vi "HMI Pop Up Alpha KB.vi"(4 "Password Display (F)":bool, 5 "Hide OVR Key (T)":bool, 6 "Max Length (70)":i32=70, 8 "error in (no error)":errorcluster, 10 "String In":string, 11 "Message In":string) -> (0 "error out":errorcluster, 1 "Canceled":bool, 2 "String Out":string)   [LabVIEW 2015]
doc: "Name: Pop Up Keyboard\nAuthor: Georges Janveau, Columbia Forest Products\n\nDESCRIPTION\nSimulates an alphanumeric keyboard intended to be used on a touchscreen PC. The input control can be set for standard or password display. The OVR key can be shown or hidden.\n\nINPUTS\nMessage In - Optional message displayedin the title bar.\nString In - Sets the initial value of the edit box.\nPassword Display (F) - Sets standard or password display.\nHide OVR Key (T) - Hides or displays the OVR key button.\nMax Length (255) - Sets the maximum length allowed in the edit box.\n\nOUTPUTS\nString Out - Result (will contain String In if the user cancels).\nCanceled - True if the user cancels.\n\n----------------------------------------------------------------------------------------------------------------"
uses:
  srv_label_inspection_line2-3-4-5/Encoder - PLC SR - MF - Image Buffer/Version2/Src/OGN_SRV_PHC_SUBVI/OGN_SRV_PHC_UI/Keyboard/Driver Commands.ctl
panel:
  out "Caps on":bool
  in  "Shift 2":bool
  in  "<\n,":bool
  in  "?\n/":bool
  in  ">\n.":bool
  in  "M\nm":bool
  in  "N\nn":bool
  in  "B\nb":bool
  in  "V\nv":bool
  in  "C\nc":bool
  in  "X\nx":bool
  in  "Z\nz":bool
  in  "\"\n'":bool
  in  ":\n;":bool
  in  "L\nl":bool
  in  "K\nk":bool
  in  "J\nj":bool
  in  "H\nh":bool
  in  "G\ng":bool
  in  "F\nf":bool
  in  "D\nd":bool
  in  "S\ns":bool
  in  "A\na":bool
  in  "}\n]":bool
  in  "{\n[":bool
  in  "|\n\\":bool
  in  "+\n=":bool
  in  "_\n-":bool
  in  "P\np":bool
  in  "O\no":bool
  in  "I\ni":bool
  in  "U\nu":bool
  in  "Y\ny":bool
  in  "T\nt":bool
  in  "R\nr":bool
  in  "E\ne":bool
  in  "W\nw":bool
  in  ")\n0":bool
  in  "(\n9":bool
  in  "*\n8":bool
  in  "&\n7":bool
  in  "^\n6":bool
  in  "%\n5":bool
  in  "$\n4":bool
  in  "#\n3":bool
  in  "@\n2":bool
  in  "!\n1":bool
  in  "Q\nq":bool
  in  "Right":bool
  in  "Left":bool
  in  "Over Write":bool
  in  "Ok":bool
  in  "Cancel":bool
  in  "Space":bool
  in  "Shift":bool
  in  "CAPS":bool
  in  "Text":string
  in  "Backspace":bool
  # "Inputs"
  # "Outputs"
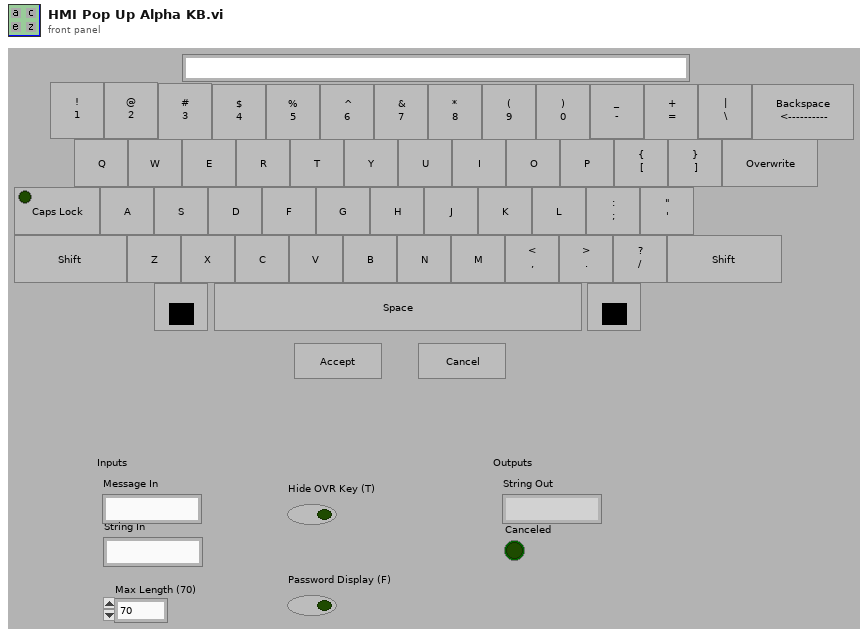
[diagram p1: front panel]
types:
  T1 = typedef "Driver Commands.ctl" = enum16{"No Command", "Initialize", "Add Character", "Replace Charcter", "Delete Character", "Move Left", "Move Right", "Update Edit Position"}
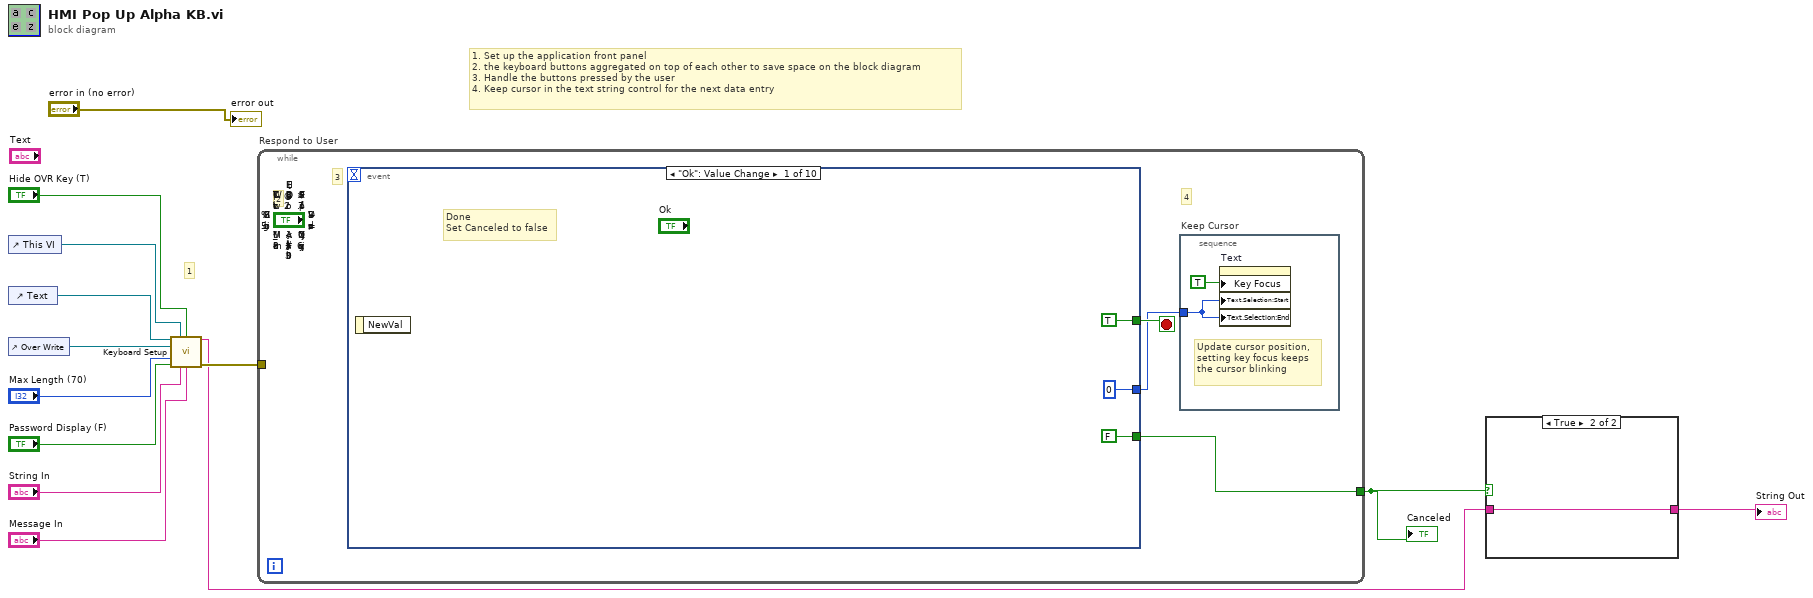
[diagram p0: block diagram]
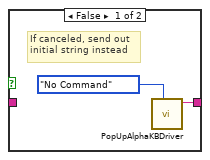
[diagram p2: hidden frame]
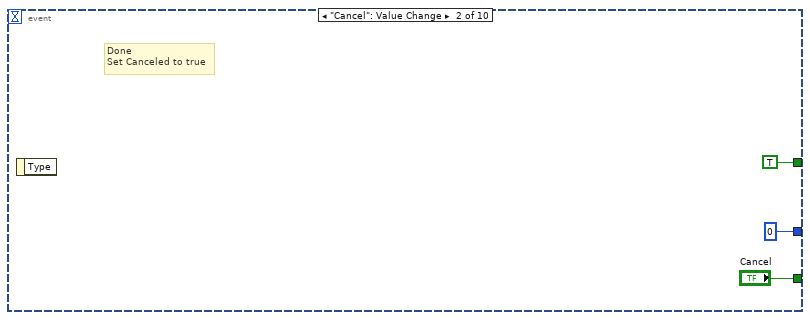
[diagram p3: hidden frame]
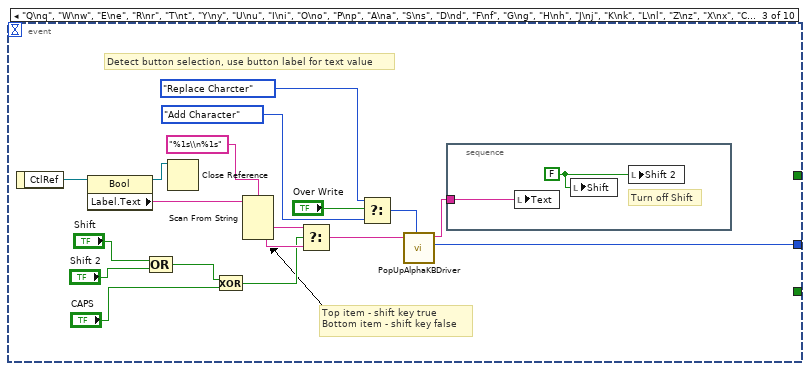
[diagram p4: hidden frame]
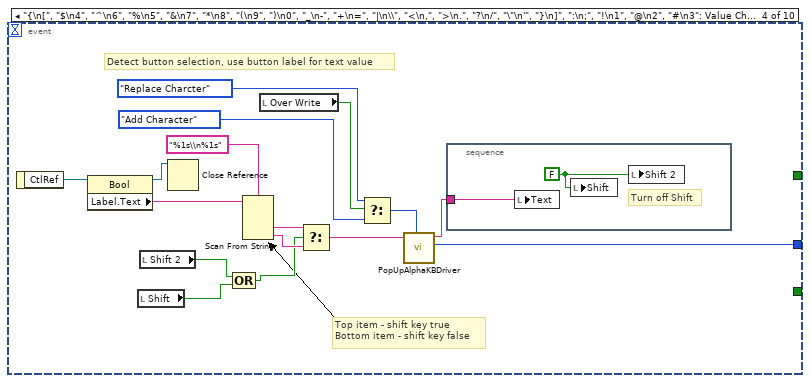
[diagram p5: hidden frame]
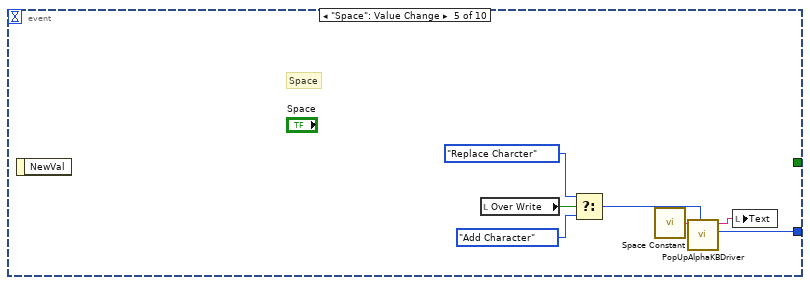
[diagram p6: hidden frame]
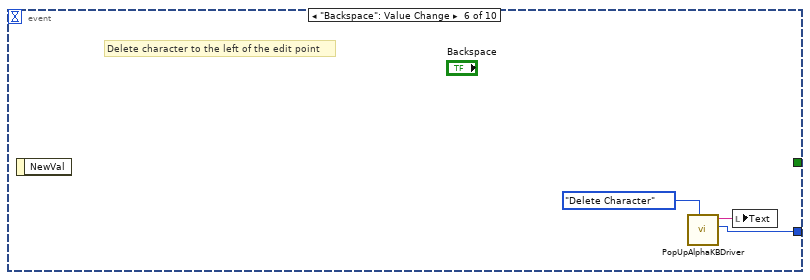
[diagram p7: hidden frame]
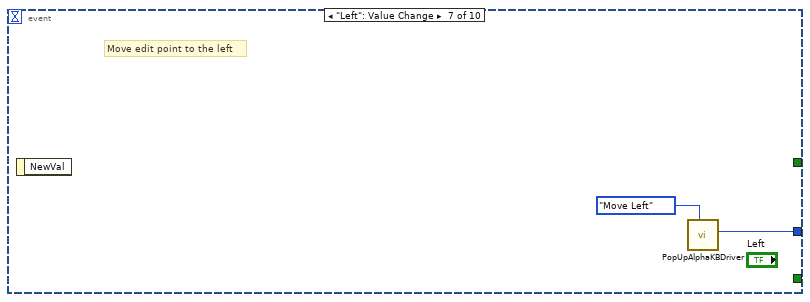
[diagram p8: hidden frame]
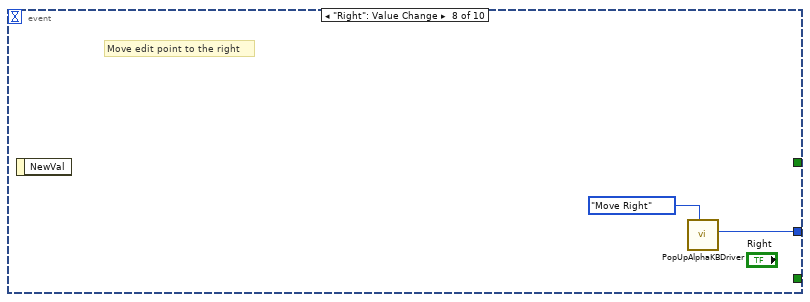
[diagram p9: hidden frame]
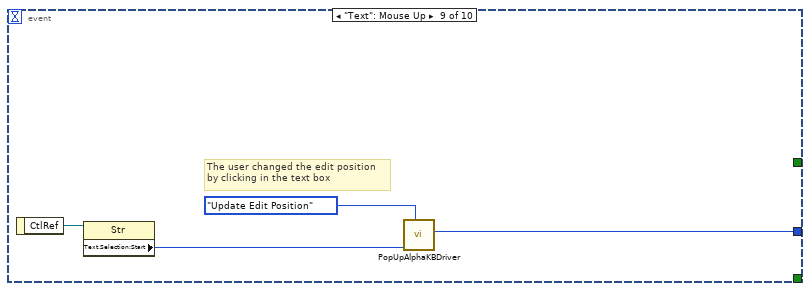
[diagram p10: hidden frame]
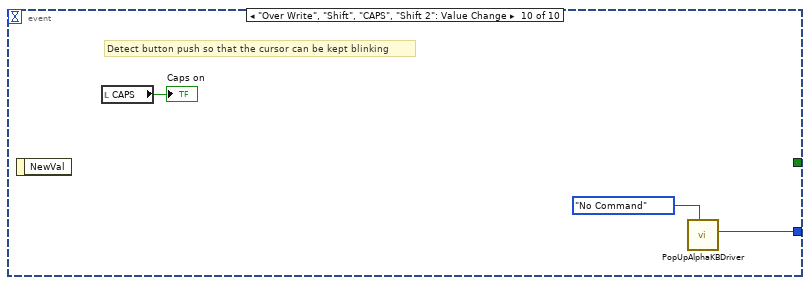
[diagram p11: hidden frame]
diagram:
  # "1. Set up the application front panel\n2. the keyboard buttons aggregated on top of each other to save space on the block diagram\n3. Handle the buttons pressed by the user\n4. Keep cursor in the text string control for the next data entry"
  # "1"
  n1 = control-ref of="This VI"() -> (w6:refnum<vi>)
  n2 = control-ref of="Text"() -> (w10:refnum<vi>)
  n3 = control-ref of="Over Write"() -> (w9:refnum<vi>)
  n4 = call "Keyboard Setup.vi"("String in"=w10, "This VI"=w6, "Hide OVR Key (T)"="Hide OVR Key (T)", "reference in"=w9, "Max Length (70)"="Max Length (70)", "Password Display (F)"="Password Display (F)", "String In"="String In", "Message In"="Message In") -> ("String Out"=w3:string, "error out"=w4:errorcluster)  [unwired: 6 in]
  n5 = while "Respond to User" {
    tunnel: [w14] -> w2
    tunnel: w4 -> [_]
    stop <- w16 stop-if-true
    # "4"
    # "2"
    # "3"
    n6 = event shown="[0] \"Ok\": Value Change" {
      selector: _ -> [_ _ _ _ _ _ _ _ _ _]
      dyn-events: _ -> [_ _ _ _ _ _ _ _ _ _]
      timeout: _ -> [_ _ _ _ _ _ _ _ _ _]
      tunnel: [TRUE TRUE _ _ _ _ _ _ _ _] -> w16
      tunnel: [0 ("Edit Position") 0 ("Edit Position") w32 w50 w65 w71 w74 w75 w77 w82] -> w15
      tunnel: [FALSE ("Cancel") "Cancel" _ _ _ _ _ _ _ _] -> w14
      event "Ok": Value Change {
        # "Done\nSet Canceled to false"
        n7 = event-data() -> ()  [unwired: 1 in, 1 out]
      }
      event "Cancel": Value Change {
        # "Done\nSet Canceled to true"
        n8 = event-data() -> ()  [unwired: 1 in, 1 out]
      }
      event "Q\nq", "W\nw", "E\ne", "R\nr", "T\nt", "Y\ny", "U\nu", "I\ni", "O\no", "P\np", "A\na", "S\ns", "D\nd", "F\nf", "G\ng", "H\nh", "J\nj", "K\nk", "L\nl", "Z\nz", "X\nx", "C\nc", "V\nv", "B\nb", "N\nn", "M\nm": Value Change {
        # "Top item - shift key true\nBottom item - shift key false"
        # "Detect button selection, use button label for text value"
        n9 = event-data() -> ("CtlRef"=w39:refnum<vi>)  [unwired: 1 in]
        n10 = property class="Bool"(reference=w39) -> (reference out=w37:refnum<vi>, "Label.Text"=w38:string)  [unwired: 1 in, 1 out]
        n11 = Compound Arithmetic op=OR("Shift", "Shift 2") -> (w27:bool)
        n12 = Close Reference(reference=w37) -> ()  [unwired: 1 in, 1 out]
        n13 = Exclusive Or(1:"CAPS", 2:w27) -> (0:w25:bool)
        n14 = Scan From String(format string="%1s\\n%1s", input string=w38) -> (output 1=w41:string, output 2=w40:string)  [unwired: 4 in, 3 out]
        n15 = Select(t=w41, s=w25, f=w40) -> (s? t:f=w36:string)
        n16 = Select(t=Driver_Commands."Replace Charcter" ("Driver Commands"), s="Over Write", f=Driver_Commands."Add Character" ("Driver Commands")) -> (s? t:f=w35:T1)
        n17 = call "PopUpAlphaKBDriver.vi"("Driver Commands"=w35, "Character"=w36) -> ("Edit Position"=w32:i32, "String Out"=w30:string)  [unwired: 8 in]
        n18 = stacked-sequence {
          tunnel: w30 -> [w44]
          frame #0 {
            w43 = FALSE ("Shift")
            # "Turn off Shift"
            n19 = local write "Text"(w44) -> ()
            n20 = local write "Shift"(w43) -> ()
            n21 = local write "Shift 2"(w43) -> ()
          }
        }
      }
      event "{\n[", "$\n4", "^\n6", "%\n5", "&\n7", "*\n8", "(\n9", ")\n0", "_\n-", "+\n=", "|\n\\", "<\n,", ">\n.", "?\n/", "\"\n'", "}\n]", ":\n;", "!\n1", "@\n2", "#\n3": Value Change {
        # "Top item - shift key true\nBottom item - shift key false"
        # "Detect button selection, use button label for text value"
        n22 = event-data() -> ("CtlRef"=w57:refnum<vi>)  [unwired: 1 in]
        n23 = property class="Bool"(reference=w57) -> (reference out=w55:refnum<vi>, "Label.Text"=w56:string)  [unwired: 1 in, 1 out]
        n24 = local read "Shift"() -> (w48:bool)
        n25 = local read "Shift 2"() -> (w47:bool)
        n26 = Close Reference(reference=w55) -> ()  [unwired: 1 in, 1 out]
        n27 = Compound Arithmetic op=OR(w47, w48) -> (w45:bool)
        n28 = Scan From String(format string="%1s\\n%1s", input string=w56) -> (output 1=w59:string, output 2=w58:string)  [unwired: 4 in, 3 out]
        n29 = local read "Over Write"() -> (w46:bool)
        n30 = Select(t=w59, s=w45, f=w58) -> (s? t:f=w54:string)
        n31 = Select(t=Driver_Commands."Replace Charcter" ("Driver Commands"), s=w46, f=Driver_Commands."Add Character" ("Driver Commands")) -> (s? t:f=w53:T1)
        n32 = call "PopUpAlphaKBDriver.vi"("Driver Commands"=w53, "Character"=w54) -> ("Edit Position"=w50:i32, "String Out"=w49:string)  [unwired: 8 in]
        n33 = stacked-sequence {
          tunnel: w49 -> [w62]
          frame #0 {
            w61 = FALSE ("Shift")
            # "Turn off Shift"
            n34 = local write "Text"(w62) -> ()
            n35 = local write "Shift"(w61) -> ()
            n36 = local write "Shift 2"(w61) -> ()
          }
        }
      }
      event "Space": Value Change {
        # "Space"
        n37 = event-data() -> ()  [unwired: 1 in, 1 out]
        n38 = local read "Over Write"() -> (w63:bool)
        n39 = Select(t=Driver_Commands."Replace Charcter" ("Driver Commands"), s=w63, f=Driver_Commands."Add Character" ("Driver Commands")) -> (s? t:f=w66:T1)
        n40 = call <vilib>:"Space Constant.vi"() -> ("String"=w69:string)
        n41 = call "PopUpAlphaKBDriver.vi"("Driver Commands"=w66, "Character"=w69) -> ("Edit Position"=w65:i32, "String Out"=w64:string)  [unwired: 8 in]
        n42 = local write "Text"(w64) -> ()
      }
      event "Backspace": Value Change {
        # "Delete character to the left of the edit point"
        n43 = event-data() -> ()  [unwired: 1 in, 1 out]
        n44 = call "PopUpAlphaKBDriver.vi"("Driver Commands"=Driver_Commands."Delete Character") -> ("Edit Position"=w71:i32, "String Out"=w70:string)  [unwired: 9 in]
        n45 = local write "Text"(w70) -> ()
      }
      event "Left": Value Change {
        # "Move edit point to the left"
        n46 = event-data() -> ()  [unwired: 1 in, 1 out]
        n47 = call "PopUpAlphaKBDriver.vi"("Driver Commands"=Driver_Commands."Move Left") -> ("Edit Position"=w74:i32)  [unwired: 9 in, 1 out]
      }
      event "Right": Value Change {
        # "Move edit point to the right"
        n48 = event-data() -> ()  [unwired: 1 in, 1 out]
        n49 = call "PopUpAlphaKBDriver.vi"("Driver Commands"=Driver_Commands."Move Right") -> ("Edit Position"=w75:i32)  [unwired: 9 in, 1 out]
      }
      event "Text": Mouse Up {
        # "The user changed the edit position\nby clicking in the text box"
        n50 = event-data() -> ("CtlRef"=w80:refnum<vi>)  [unwired: 1 in]
        n51 = property class="Str"(reference=w80) -> ("Text.Selection:Start"=w79:u32)  [unwired: 1 in, 2 out]
        n52 = call "PopUpAlphaKBDriver.vi"("Driver Commands"=Driver_Commands."Update Edit Position", "New Edit Position"=w79) -> ("Edit Position"=w77:i32)  [unwired: 8 in, 1 out]
      }
      event "Over Write", "Shift", "CAPS", "Shift 2": Value Change {
        # "Detect button push so that the cursor can be kept blinking"
        n53 = event-data() -> ()  [unwired: 1 in, 1 out]
        n54 = local read "CAPS"() -> (→"Caps on":bool)
        n55 = call "PopUpAlphaKBDriver.vi"("Driver Commands"=Driver_Commands."No Command") -> ("Edit Position"=w82:i32)  [unwired: 9 in, 1 out]
      }
    }
    n56 = stacked-sequence "Keep Cursor" {
      tunnel: w15 -> [w17]
      frame #0 {
        # "Update cursor position,\nsetting key focus keeps\nthe cursor blinking"
        n57 = property on="Text" class="Str"("Key Focus"=TRUE, "Text.Selection:Start"=w17, "Text.Selection:End"=w17) -> ()  [unwired: 2 in, 2 out]
      }
    }
  }
  "Canceled" <- w2
  n58 = case shown="True" w2 {
    tunnel: [w84 w86] -> w5
    tunnel: w3 -> [_ w86]
    frame False {
      # "If canceled, send out\ninitial string instead"
      n59 = call "PopUpAlphaKBDriver.vi"("Driver Commands"=Driver_Commands."No Command") -> ("String Out"=w84:string)  [unwired: 9 in, 1 out]
    }
    frame True {
    }
  }
  "String Out" <- w5
  "error out" <- "error in (no error)"
